vi "dfd_Validate Params for One Point Notch Peak Design by Q.vi"(6 "fs [Hz]":dbl=1.0 format="%.2f", 8 "error in (no error)":errorcluster, 10 "Q factor":dbl=3.0 format="%.2f", 11 "f0 [Hz]":dbl format="%.2f") -> (0 "error out":errorcluster, 1 "normalized bandwidth":dbl format="%.2f", 3 "normalized f0":dbl format="%.2f")   [LabVIEW 2017, in "NI_DigFilter_Design.lvlib"]
uses:
  <vilib>/addons/Digital Filter Design/NI_DigFilter_Design.lvlib
  <vilib>/addons/Digital Filter Design/_Misc.llb/dfd_Error Handlers (Multiple).vi
  <vilib>/addons/Digital Filter Design/NI_DigFilterLicensed.lvlib
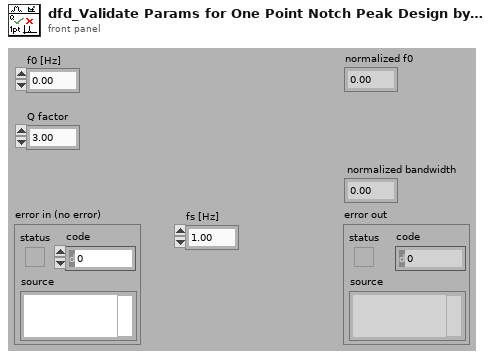
[diagram p1: front panel]
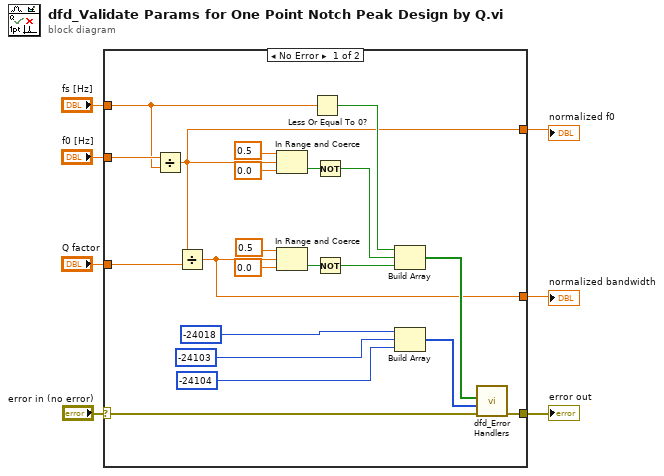
[diagram p0: block diagram]
diagram:
  n1 = case shown="No Error" "error in (no error)" {
    selector: "error in (no error)" -> [w26 w29]
    tunnel: "Q factor" -> [w10 _]
    tunnel: "f0 [Hz]" -> [w28 _]
    tunnel: [w27 w29] -> w5
    tunnel: "fs [Hz]" -> [w23 _]
    tunnel: [w11 _] -> w3
    tunnel: [w16 _] -> w2
    frame No Error {
      n2 = Divide(x=w28, y=w23) -> (x/y=w11:dbl)
      n3 = Divide(x=w11, y=w10) -> (x/y=w16:dbl)
      n4 = In Range and Coerce(upper limit=0.5 ("y"), x=w11, lower limit=0.0 ("y")) -> (In Range?=w20:bool)  [unwired: 1 out]
      n5 = In Range and Coerce(upper limit=0.5 ("y"), x=w16, lower limit=0.0 ("y")) -> (In Range?=w17:bool)  [unwired: 1 out]
      n6 = Less Or Equal To 0?(x=w23) -> (x <= 0?=w15:bool)
      n7 = Not(x=w20) -> (.not. x?=w14:bool)
      n8 = Not(x=w17) -> (.not. x?=w9:bool)
      n9 = Build Array(w15, w14, w9) -> (w25:bool[])
      n10 = Build Array(-24018 ("ERR_FS_LE_ZERO"), -24103 ("ERR_F0BYQ_RANGE_WRONG"), -24104 ("ERR_Q_RANGE_WRONG")) -> (w24:i32[])
      n11 = call-poly <vilib>:"dfd_Error Handlers.vi"("error in (no error)"=w26, "error sources"=w24, "condition failed?"=w25) -> ("error out"=w27:errorcluster)  [unwired: 8 out]
    }
    frame Error {
    }
  }
  "normalized bandwidth" <- w2
  "normalized f0" <- w3
  "error out" <- w5
